vi "CallChainOptionsMapFGV.vi"(7 "Action":T1, 8 "error in (no error)":errorcluster, 10 "BlueJSONTextSerializer (Add)":refnum<class "BlueJSONTextSerializer.lvclass">, 11 "CloneID":string) -> (0 "error out":errorcluster, 1 "key not found?":bool, 2 "BlueJSONTextSerializer (Read, Remove)":refnum<class "BlueJSONTextSerializer.lvclass">)   [LabVIEW 2019]
uses:
  BlueJSONTextSerializer.lvclass
  OptionsFGVAction.ctl
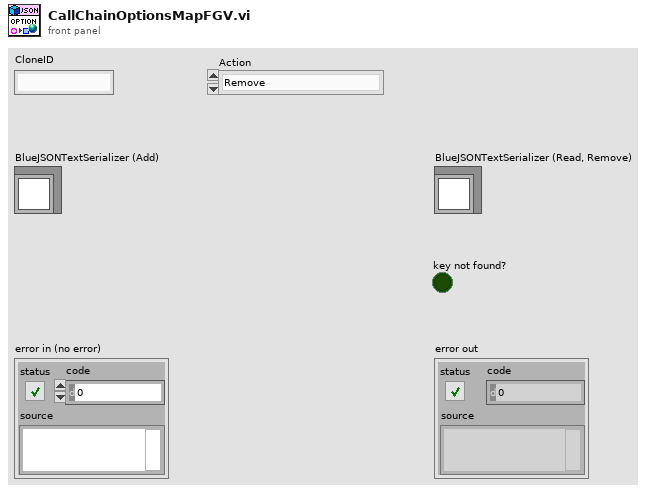
[diagram p1: front panel]
types:
  T1 = typedef "BlueJSONTextSerializer.lvlib/BlueJSONTextSerializer.lvclass/OptionsFGVAction.ctl" = enum16{"Remove", "Read", "Add"}
  T2 = map{string, refnum<class "BlueJSONTextSerializer.lvclass">}
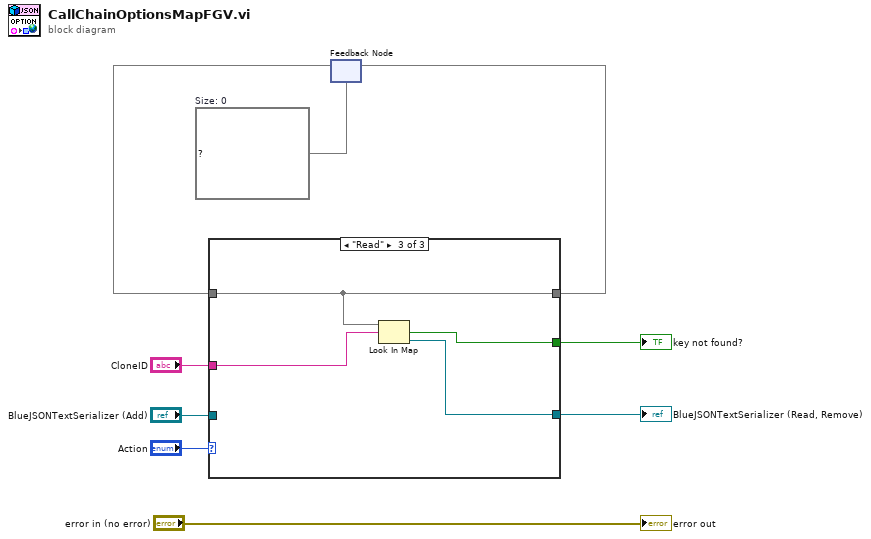
[diagram p0: block diagram]
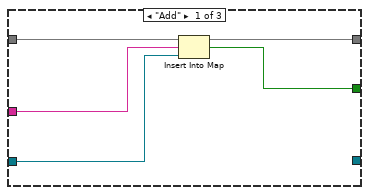
[diagram p2: hidden frame]
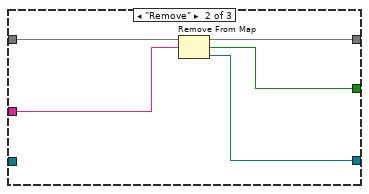
[diagram p3: hidden frame]
diagram:
  w9 = T2 {}  # Size: 0
  n1 = feedback #1(w9) -> (w8:T2)
  n2 = case shown="\"Read\"" "Action" {
    tunnel: w8 -> [w14 w19 w23]
    tunnel: "CloneID" -> [w13 w17 w22]
    tunnel: "BlueJSONTextSerializer (Add)" -> [w11 _ _]
    tunnel: [w12 w18 w23] -> w5
    tunnel: [_ w15 w21] -> w1
    tunnel: [w10 w16 w20] -> w4
    frame "Add" {
      n3 = Insert Into Map(map in=w14, key=w13, value=w11) -> (map out=w12:T2, key already included?=w10:bool)  [unwired: 1 out]
    }
    frame "Remove" {
      n4 = Remove From Map(10:w17, 11:w19) -> (1:w15:refnum<class "BlueJSONTextSerializer.lvclass">, 2:w16:bool, 3:w18:T2)
    }
    frame "Read" {
      n5 = Look In Map(map=w23, key=w22) -> (key not found?=w20:bool, value=w21:refnum<class "BlueJSONTextSerializer.lvclass">)  [unwired: 1 in]
    }
  }
  "key not found?" <- w4
  "BlueJSONTextSerializer (Read, Remove)" <- w1
  n6 = feedback-in #1(w5) -> ()
  "error out" <- "error in (no error)"
